vi "Write column.vi"(8 "error in (no error)":errorcluster, 10 "column":i32, 11 "CellValueChanged in":refnum<class "CellDirtyStateChanged.lvclass">) -> (0 "error out":errorcluster, 3 "CellValueChanged out":refnum<class "CellDirtyStateChanged.lvclass">)   [LabVIEW 2013, in "DataGrid.lvlib" / "CellDirtyStateChanged.lvclass"]
uses:
  CellDirtyStateChanged.lvclass
  CellDirtyStateChanged.lvclass/CellDirtyStateChanged.ctl
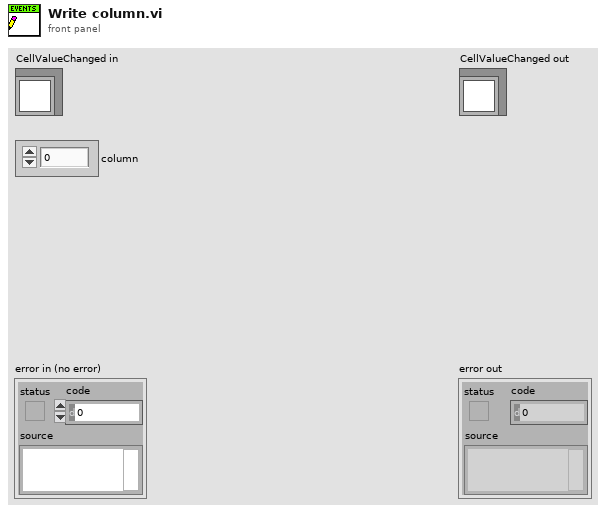
[diagram p1: front panel]
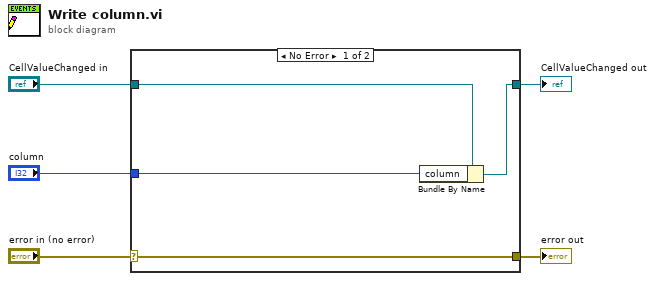
[diagram p0: block diagram]
diagram:
  n1 = case shown="No Error" "error in (no error)" {
    selector: "error in (no error)" -> [w9 w10]
    tunnel: [w9 w10] -> w4
    tunnel: [w7 w11] -> w2
    tunnel: "CellValueChanged in" -> [w8 w11]
    tunnel: "column" -> [w6 _]
    frame No Error {
      n2 = Bundle By Name(cluster=w8, "column"=w6) -> (w7:refnum<class "CellDirtyStateChanged.lvclass">)
    }
    frame Error {
    }
  }
  "error out" <- w4
  "CellValueChanged out" <- w2
